vi "ManualTresholdControlNOGEN.vi"() -> ()   [LabVIEW 2012]
uses:
  <vilib>/Utility/NIReport.llb/NI_report.lvclass
  <vilib>/Utility/NIReport.llb/HTML/NI_HTML.lvclass
panel:
  out "IPR_count":u32
  in  "Channel":i8=6
  in  "Instrument VISA in":T1={"AWG VISA"="AgilentGenerator1", "Oscilloscope  VISA "="AgilentOsciloscope", "Integration Board IP"="172.16.17.47", "connection ID"=refnum, "report out"=refnum, "report file path"=path "C:/Documents and Settings/CTA_LAB01/Desktop/L0_Asic/L0 Asic Test Data"}
  in  "Treshold":i16(slide)=557 min=0 max=1000 scale=0.0..1000.0
  in  "stop":bool
  out "error out":errorcluster
  in  "error in":errorcluster
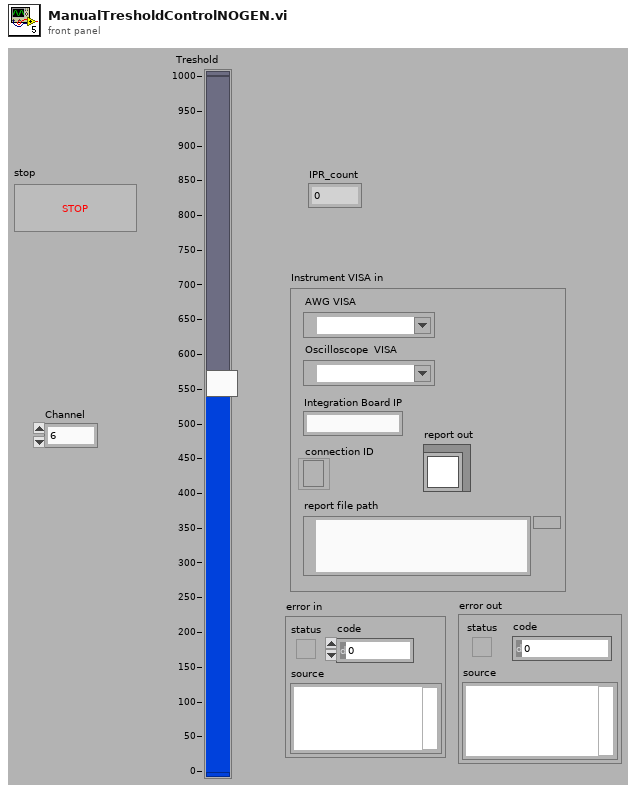
[diagram p1: front panel]
types:
  T1 = cluster{"AWG VISA":refnum<visa-resource-name>, "Oscilloscope  VISA ":refnum<visa-resource-name>, "Integration Board IP":string, "connection ID":refnum<k5>, "report out":refnum<class "NI_report.lvclass">, "report file path":path}
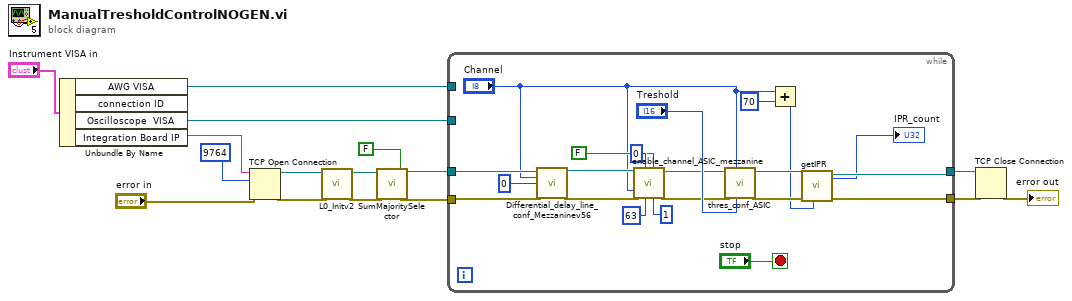
[diagram p0: block diagram]
diagram:
  n1 = Unbundle By Name("Instrument VISA in") -> ("AWG VISA"=w2:refnum<visa-resource-name>, "Oscilloscope  VISA"=w3:refnum<visa-resource-name>, "Integration Board IP"=w11:string)  [unwired: 1 out]
  n2 = TCP Open Connection(address=w11, remote port or service name=u16 9764, error in (no error)="error in") -> (connection ID=w10:refnum<k5>, error out=w9:errorcluster)  [unwired: 2 in]
  n3 = call "L0_Initv2.vi"("error in"=w9, "connection ID in"=w10) -> ("error out"=w8:errorcluster, "connection ID out"=w7:refnum<k5>)  [unwired: 8 in]
  n4 = call "SumMajoritySelector.vi"("On Sum\nOff Majority"=FALSE ("On Sum\nOff Majority"), "error in (no error)"=w8, "connection ID"=w7) -> ("error out"=w5:errorcluster, "connection ID out"=w6:refnum<k5>)  [unwired: 5 in]
  n5 = while {
    tunnel: [w24] -> w14
    tunnel: [w22] -> w13
    tunnel: w5 -> [w17]
    tunnel: w6 -> [w27]
    tunnel: w3 -> [_]
    tunnel: w2 -> [_]
    stop <- "stop" stop-if-true
    n6 = call "Differential_delay_line_conf_Mezzaninev56.vi"("connection ID"=w27, "channel"="Channel", "Delay value"=u16 0, "error in (no error)"=w17) -> ("connection ID out"=w32:refnum<k5>, "error out 2"=w34:errorcluster)  [unwired: 4 in, 6 out]
    n7 = call "enable_channel_ASIC_mezzanine.vi"("Clip_sel_b"=u32 1, "maj/sum"=FALSE, "Ib_clipVb"=u32 63, "Att gain"=u32 0, "error in"=w34, "Channel"="Channel", "connection ID"=w32) -> ("error out"=w33:errorcluster, "connection ID out"=w31:refnum<k5>)  [unwired: 2 in, 1 out]
    n8 = call "thres_conf_ASIC.vi"("threshold"="Treshold", "Ring"="Channel", "error out 3"=w33, "connection ID"=w31) -> ("error out 2"=w25:errorcluster, "connection ID out"=w23:refnum<k5>)  [unwired: 4 in, 2 out]
    n9 = Add(x="Channel", y=i8 70) -> (x+y=w18:i8)
    n10 = call "getIPR.vi"("Address"=w18, "error in"=w25, "connection ID"=w23) -> ("error out"=w24:errorcluster, "connection ID out"=w22:refnum<k5>, "IPR_count"=→"IPR_count":u32)  [unwired: 5 in, 1 out]
  }
  n11 = TCP Close Connection(connection ID=w13, error in (no error)=w14) -> (error out=→"error out":errorcluster)  [unwired: 1 in, 1 out]
